vi "4 Sync - Shared Time Base No Drift.vi"() -> ()   [LabVIEW 2023]
doc: "This example demonstrates how to acquire a single buffer of voltage measurements using a DAQmx device.\n\nFor instructions on how to connect your signals to the DAQ device, refer to your device documentation."
uses:
  <vilib>/DAQmx/create/channels.llb/DAQmx Create Channel (AI-Voltage-Basic).vi
  <vilib>/DAQmx/configure/timing.llb/DAQmx Timing (Sample Clock).vi
  <vilib>/DAQmx/read.llb/DAQmx Read (Analog Wfm 1Chan NSamp).vi
  <resource>/objmgr/daqmx.rc
  <vilib>/DAQmx/create/channels.llb/DAQmx Create Channel (CO-Pulse Generation-Frequency).vi
  <vilib>/DAQmx/configure/timing.llb/DAQmx Timing (Implicit).vi
panel:
  in  "Device 2: Sample Clock Source":tag="/cDAQ9189-2628AACMod5/PFI4"
  in  "stop":bool
  in  "Sample Clock Output: Terminal":tag="/MIODAQ/PFI2"
  in  "Square Wave Output: Terminal":tag="/MIODAQ/PFI0"
  in  "Square Wave Output: Source":tag="MIODAQ/ctr0"
  out "Skew":dbl=-1.072865529480623
  in  "Device 2: Analog Input Channel":tag="cDAQ9189-2628AACMod1/ai0"
  out "Waveform Graph":waveform(dbl)[](graph)=[{"t0"=timestamp(3851425488.627929 s since 1904-01-01), "dt"=9.999999999999972e-06, "Y"=array[100000 elements], "attributes"=variant("NI_ChannelName"=variant(string "MIODAQ/ai0"), "NI_UnitDescription"=variant(string "Volts"))}, {"t0"=timestamp(3851425488.628186 s since 1904-01-01), "dt"=9.999999999999972e-06, "Y"=array[100000 elements], "attributes"=variant("NI_ChannelName"=variant(string "cDAQ9189-2628AACMod1/ai0"), "NI_UnitDescription"=variant(string "Volts"))}]
  in  "Device 1 & 2: Sample Rate":dbl=100000.0
  in  "Device 1: Sample Clock Source":tag="OnboardClock"
  in  "Device 1: Analog Input Channel":tag="MIODAQ/ai0"
  # "Channel Settings"
  # "Acquired Data"
  # "Timing Settings"
  # "Output Signal Settings"
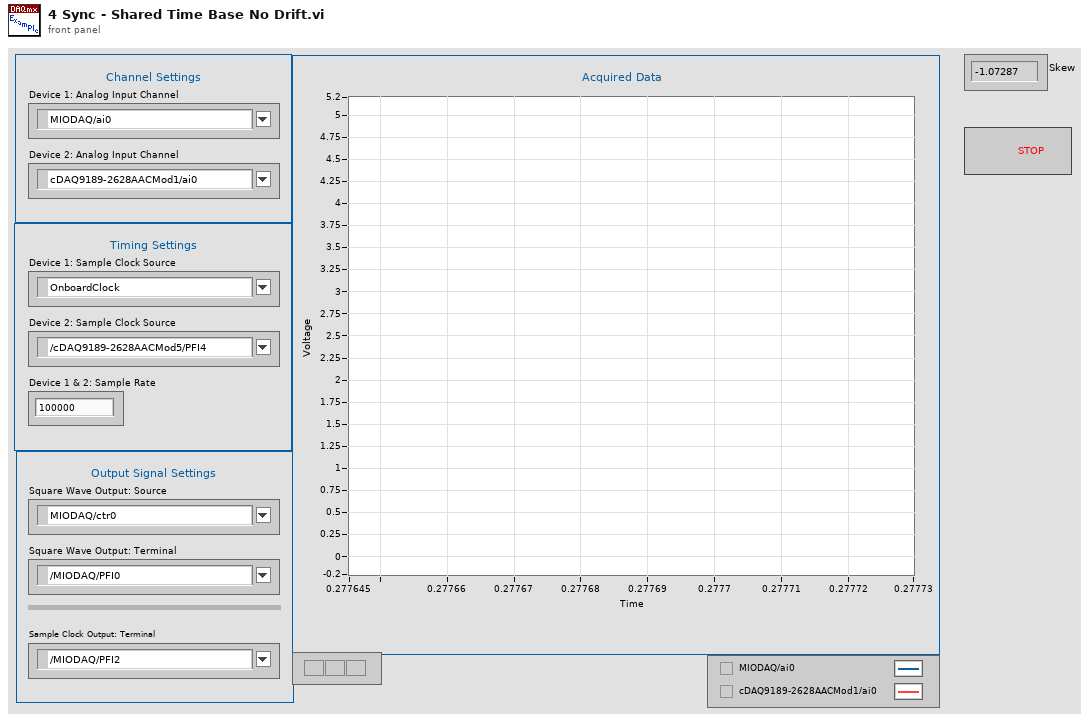
[diagram p1: front panel]
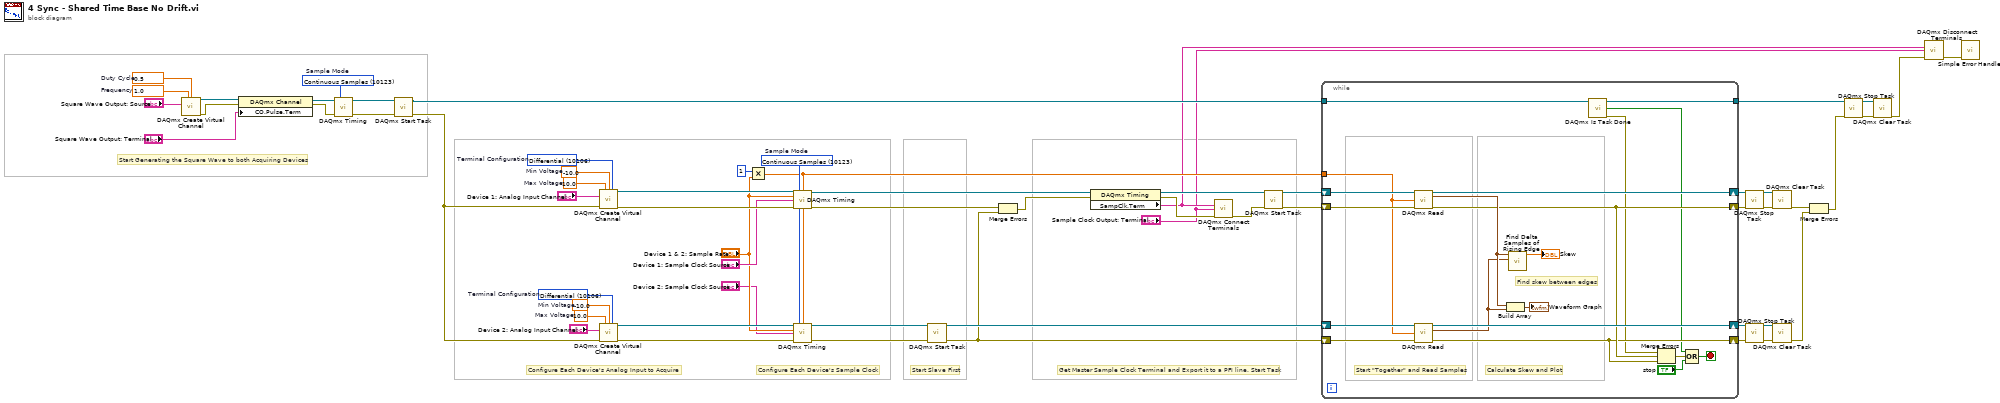
[diagram p0: block diagram]
diagram:
  w38 = 10.0  # Max Voltage
  w37 = -10.0  # Min Voltage
  w36 = 10106 items=["default"=-1, "RSE"=10083, "NRSE"=10078, "Differential"=10106, "Pseudodifferential"=12529]  # Terminal Configuration
  w42 = 10.0  # Max Voltage
  w43 = -10.0  # Min Voltage
  w44 = 10106 items=["default"=-1, "RSE"=10083, "NRSE"=10078, "Differential"=10106, "Pseudodifferential"=12529]  # Terminal Configuration
  w26 = 10123 items=["Finite Samples"=10178, "Continuous Samples"=10123, "Hardware Timed Single Point"=12522]  # Sample Mode
  w58 = 1.0  # Frequency
  w59 = 0.5  # Duty Cycle
  w51 = 10123 items=["Finite Samples"=10178, "Continuous Samples"=10123, "Hardware Timed Single Point"=12522]  # Sample Mode
  # "Get Master Sample Clock Terminal and Export it to a PFI line. Start Task"
  # "Start Slave First"
  # "Configure Each Device's Sample Clock"
  # "Configure Each Device's Analog Input to Acquire"
  # "Start Generating the Square Wave to both Acquiring Devices"
  n1 = call-poly <vilib>:"DAQmx Create Virtual Channel.vi"("frequency"=w58, "duty cycle"=w59, "counter"="Square Wave Output: Source") -> ("task out"=w53:refnum<k21>, "error out"=w54:errorcluster)  [unwired: 11 in]
  n2 = property class="DAQmx Channel"(reference=w53, error in=w54, "CO.Pulse.Term"="Square Wave Output: Terminal") -> (reference out=w57:refnum<k21>, error out=w56:errorcluster)
  n3 = call-poly <vilib>:"DAQmx Timing.vi"("task/channels in"=w57, "sample mode"=w51, "error in"=w56) -> ("task out"=w61:refnum<k21>, "error out"=w60:errorcluster)  [unwired: 11 in]
  n4 = call <vilib>:"DAQmx Start Task.vi"("task/channels in"=w61, "error in"=w60) -> ("task out"=w18:refnum<k21>, "error out"=w9:errorcluster)  [unwired: 12 in]
  n5 = call-poly <vilib>:"DAQmx Create Virtual Channel.vi"("maximum value"=w42, "minimum value"=w43, "input terminal configuration"=w44, "physical channels"="Device 1: Analog Input Channel", "error in"=w9) -> ("task out"=w47:refnum<k21>, "error out"=w48:errorcluster)  [unwired: 9 in]
  n6 = call-poly <vilib>:"DAQmx Create Virtual Channel.vi"("maximum value"=w38, "minimum value"=w37, "input terminal configuration"=w36, "physical channels"="Device 2: Analog Input Channel", "error in"=w9) -> ("task out"=w35:refnum<k21>, "error out"=w34:errorcluster)  [unwired: 9 in]
  n7 = Multiply(x=1, y="Device 1 & 2: Sample Rate") -> (x*y=w19:dbl)
  n8 = call-poly <vilib>:"DAQmx Timing.vi"("task/channels in"=w47, "sample mode"=w26, "samples per channel"=w19, "rate"="Device 1 & 2: Sample Rate", "source"="Device 1: Sample Clock Source", "error in"=w48) -> ("task out"=w16:refnum<k21>, "error out"=w2:errorcluster)  [unwired: 8 in]
  n9 = call-poly <vilib>:"DAQmx Timing.vi"("task/channels in"=w35, "sample mode"=w26, "samples per channel"=w19, "rate"="Device 1 & 2: Sample Rate", "source"="Device 2: Sample Clock Source", "error in"=w34) -> ("task out"=w13:refnum<k21>, "error out"=w14:errorcluster)  [unwired: 8 in]
  n10 = call <vilib>:"DAQmx Start Task.vi"("task/channels in"=w13, "error in"=w14) -> ("task out"=w27:refnum<k21>, "error out"=w3:errorcluster)  [unwired: 12 in]
  n11 = Merge Errors(w2, w3) -> (w1:errorcluster)
  n12 = property class="DAQmx Timing"(reference=w16, error in=w1) -> (reference out=w15:refnum<k21>, error out=w11:errorcluster, "SampClk.Term"=w5:tag)
  n13 = call <vilib>:"DAQmx Connect Terminals.vi"("source terminal"=w5, "destination terminal"="Sample Clock Output: Terminal", "error in"=w11) -> ("error out"=w12:errorcluster)  [unwired: 12 in]
  n14 = call <vilib>:"DAQmx Start Task.vi"("task/channels in"=w15, "error in"=w12) -> ("task out"=w46:refnum<k21>, "error out"=w20:errorcluster)  [unwired: 12 in]
  n15 = while {
    shift-right: [w79] -> w39
    shift-left: w46 -> [w80]
    shift-right: [w78] -> w30
    shift-left: w27 -> [w77]
    shift-right: [w69] -> w31
    shift-left: w3 -> [w73]
    shift-right: [w70] -> w23
    shift-left: w20 -> [w72]
    tunnel: w19 -> [w71]
    tunnel: w18 -> [w65]
    tunnel: [w62] -> w17
    stop <- w66 stop-if-true
    # "Calculate Skew and Plot"
    # "Start \"Together\" and Read Samples"
    # "Find skew between edges"
    n16 = call-poly <vilib>:"DAQmx Read.vi"("task/channels in"=w80, "number of samples per channel"=w71, "error in"=w72) -> ("task out"=w79:refnum<k21>, "data"=w75:waveform(dbl), "error out"=w70:errorcluster)  [unwired: 10 in]
    n17 = call-poly <vilib>:"DAQmx Read.vi"("task/channels in"=w77, "number of samples per channel"=w71, "error in"=w73) -> ("task out"=w78:refnum<k21>, "data"=w74:waveform(dbl), "error out"=w69:errorcluster)  [unwired: 10 in]
    n18 = Build Array(w75, w74) -> (→"Waveform Graph":waveform(dbl)[])
    n19 = call "Find Delta Samples of Rising Edge.vi"("Channel 2"=w74, "Channel 1"=w75) -> ("Sample Offset"=→"Skew":dbl)  [unwired: 9 in]
    n20 = call <vilib>:"DAQmx Is Task Done.vi"("task/channels in"=w65) -> ("task out"=w62:refnum<k21>, "task done?"=w63:bool, "error out"=w64:errorcluster)  [unwired: 12 in]
    n21 = Merge Errors(w64, w70, w69) -> (w68:errorcluster)
    n22 = Compound Arithmetic op=OR(w63, w68, "stop") -> (w66:bool)
  }
  n23 = call <vilib>:"DAQmx Stop Task.vi"("task/channels in"=w39, "error in"=w23) -> ("task out"=w41:refnum<k21>, "error out"=w40:errorcluster)  [unwired: 12 in]
  n24 = call <vilib>:"DAQmx Stop Task.vi"("task/channels in"=w30, "error in"=w31) -> ("task out"=w28:refnum<k21>, "error out"=w29:errorcluster)  [unwired: 12 in]
  n25 = call <vilib>:"DAQmx Clear Task.vi"("task in"=w41, "error in"=w40) -> ("error out"=w24:errorcluster)  [unwired: 13 in]
  n26 = call <vilib>:"DAQmx Clear Task.vi"("task in"=w28, "error in"=w29) -> ("error out"=w25:errorcluster)  [unwired: 13 in]
  n27 = Merge Errors(w24, w25) -> (w8:errorcluster)
  n28 = call <vilib>:"DAQmx Stop Task.vi"("task/channels in"=w17, "error in"=w8) -> ("task out"=w49:refnum<k21>, "error out"=w50:errorcluster)  [unwired: 12 in]
  n29 = call <vilib>:"DAQmx Clear Task.vi"("task in"=w49, "error in"=w50) -> ("error out"=w7:errorcluster)  [unwired: 13 in]
  n30 = call <vilib>:"DAQmx Disconnect Terminals.vi"("source terminal"=w5, "destination terminal"="Sample Clock Output: Terminal", "error in"=w7) -> ("error out"=w6:errorcluster)  [unwired: 12 in]
  n31 = call <vilib>:"Simple Error Handler.vi"("error in (no error)"=w6) -> ()  [unwired: 4 in, 5 out]
